vi "UI.vi"(9 "Event Registration Refnum in":refnum<event-registration>) -> ()   [LabVIEW 2019]
uses:
  Type Definitions/UI.ctl
  Type Definitions/UIOscillatorParam.ctl
  Type Definitions/Sub Oscillalator Type.ctl
  Type Definitions/UIADSRParam.ctl
  Type Definitions/UILowpassParam.ctl
  Type Definitions/UITremolo.ctl
  Type Definitions/DataInOut.ctl
panel:
  out "Waveform preview":waveform(dbl)(graph)
  in  "Input data":T1={"Play sound"=FALSE, "Stop Application"=FALSE, "Oscillator"={"Waveform Type"=enum."Sine Wave", "Frequency"=856.9737569249443, "Pulse Width"=50.10820125762328, "Sub oscillator"=enum."Off"}, "VCA"={"Volume"=49.9097556730832, "A"=50, "S"=100, "R"=50, "D"=50}, "Lowpass filter"={"On / Off"=FALSE, "Cutoff"=12290.454833178042}, "Tremolo"={"On / Off"=FALSE, "Frequency"=2.677004056526059, "Rate"=0.0}} {"Tremolo"."Rate" min=0.0 max=100.0 scale=0.0..1.0; "Tremolo"."Frequency" min=0.0 max=100.0 scale=0.0..25.0; "Lowpass filter"."Cutoff" min=0.0 max=100.0 scale=20.0..20000.0; "VCA"."D" scale=1.0..100.0; "VCA"."R" scale=1.0..100.0; "VCA"."S" scale=1.0..100.0; "VCA"."A" scale=1.0..100.0; "VCA"."Volume" min=0.0 max=100.0 scale=0.0..100.0; "Oscillator"."Pulse Width" min=0.0 max=100.0 scale=0.0..100.0; "Oscillator"."Frequency" min=0.0 max=100.0 scale=20.0..20000.0}
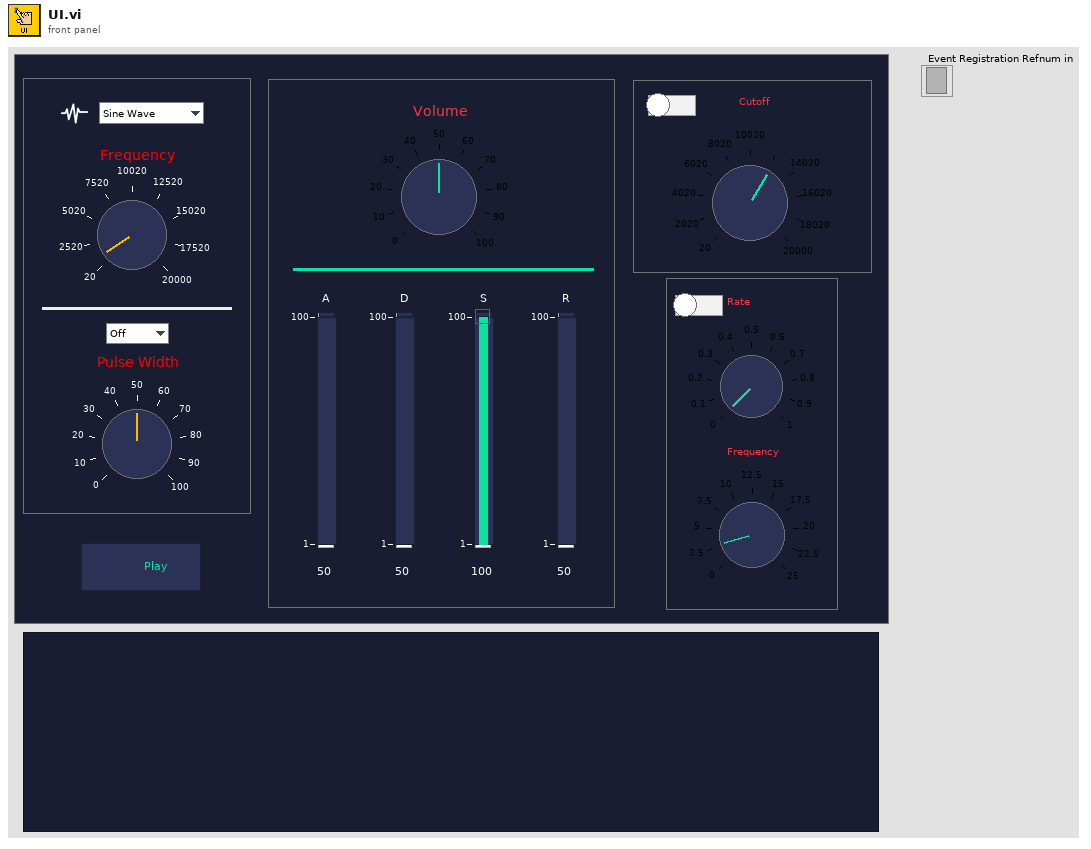
[diagram p1: front panel]
types:
  T1 = typedef "UI.ctl" = cluster{"Play sound":bool, "Stop Application":bool, "Oscillator":T2, "VCA":T4, "Lowpass filter":T5, "Tremolo":T6}
  T2 = typedef "UIOscillatorParam.ctl" = cluster{"Waveform Type":enum16{"Sine Wave", "Triangle Wave", "Square Wave", "Sawtooth Wave"}, "Frequency":dbl, "Pulse Width":dbl, "Sub oscillator":T3}
  T3 = typedef "Sub Oscillalator Type.ctl" = enum16{"Off", "One Octave", "Two Octaves"}
  T4 = typedef "UIADSRParam.ctl" = cluster{"Volume":dbl, "A":i8, "S":i8, "R":i8, "D":i8}
  T5 = typedef "UILowpassParam.ctl" = cluster{"On / Off":bool, "Cutoff":dbl}
  T6 = typedef "UITremolo.ctl" = cluster{"On / Off":bool, "Frequency":dbl, "Rate":dbl}
  T7 = typedef "DataInOut.ctl" = enum16{"Write", "Read"}
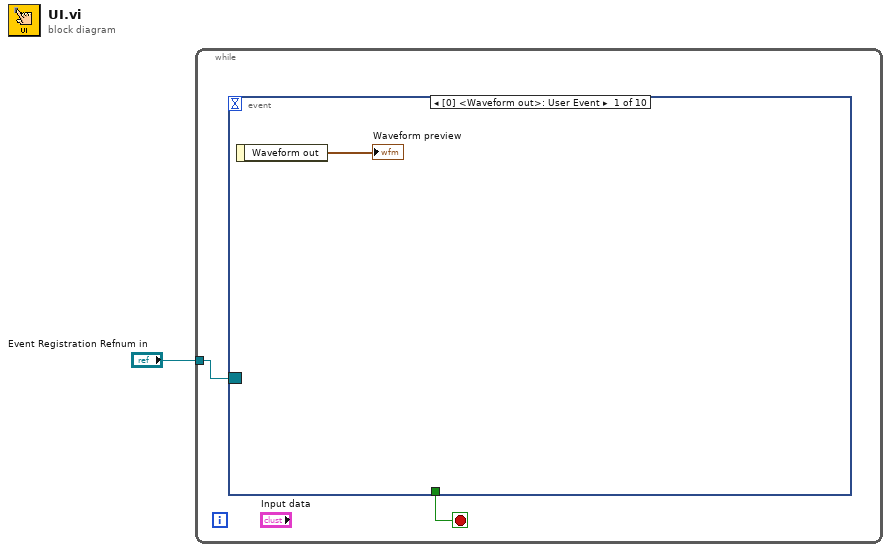
[diagram p0: block diagram]
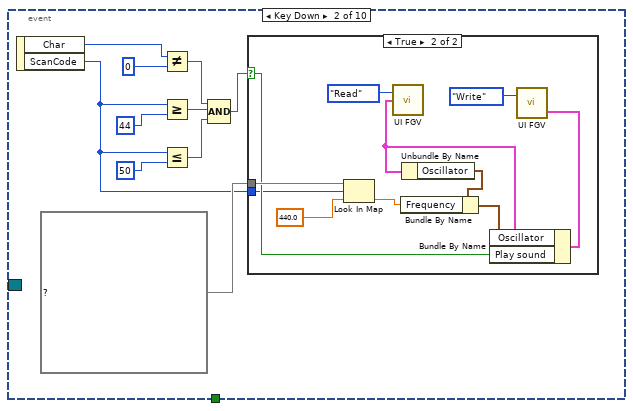
[diagram p2: hidden frame]
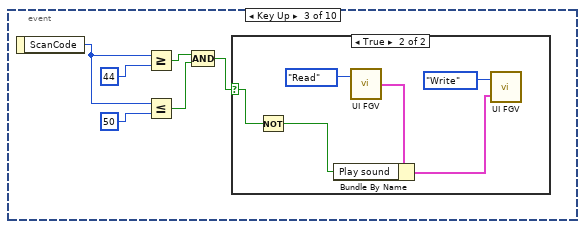
[diagram p4: hidden frame]
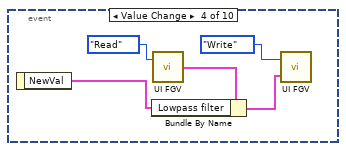
[diagram p6: hidden frame]
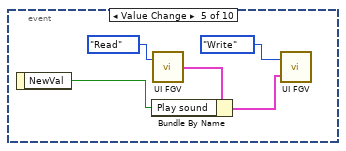
[diagram p7: hidden frame]
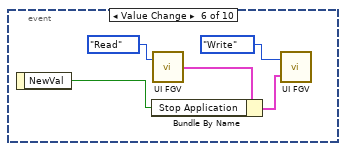
[diagram p8: hidden frame]
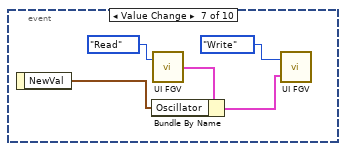
[diagram p9: hidden frame]
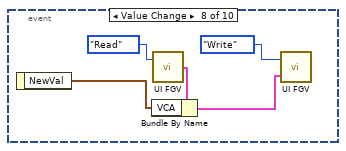
[diagram p10: hidden frame]
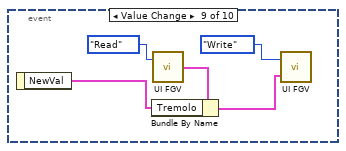
[diagram p11: hidden frame]
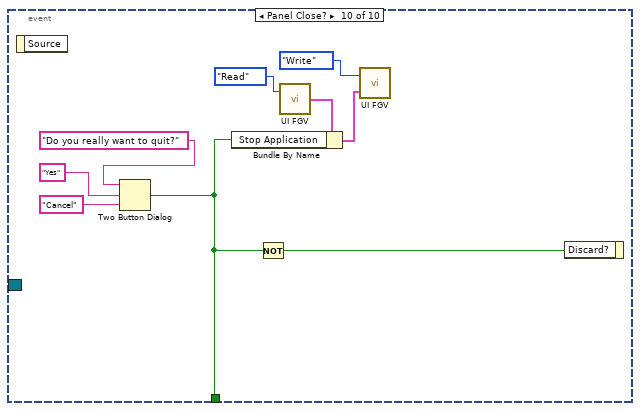
[diagram p12: hidden frame]
diagram:
  n1 = while "User Interface" {
    tunnel: "Event Registration Refnum in" -> [w3]
    stop <- w2 stop-if-true
    n2 = event shown="[0] <Waveform out>: User Event" {
      selector: w3 -> [_ _ _ _ _ _ _ _ _ _]
      dyn-events: _ -> [_ _ _ _ _ _ _ _ _ _]
      timeout: _ -> [_ _ _ _ _ _ _ _ _ _]
      tunnel: [_ _ _ _ _ _ _ _ _ w68] -> w2
      event User Event {
        n3 = event-data() -> ("Waveform out"=→"Waveform preview":waveform(dbl))  [unwired: 1 in]
      }
      event Key Down {
        n4 = event-data() -> ("Char"=w7:i16, "ScanCode"=w5:i16)  [unwired: 1 in]
        n5 = Not Equal?(x=w7, y=i16 0) -> (x != y?=w11:bool)
        n6 = Greater Or Equal?(x=w5, y=i16 44) -> (x >= y?=w10:bool)
        n7 = Less Or Equal?(x=w5, y=i16 50) -> (x <= y?=w9:bool)
        n8 = Compound Arithmetic op=AND(w11, w10, w9) -> (w6:bool)
        n9 = case shown="True" w6 {
          selector: w6 -> [_ w16]
          tunnel: map{i16, dbl} {44=261.6255653005986, 45=277.1826309768721, 46=293.66476791740763, 47=311.1269837220809, 48=329.62755691286986, 49=349.22823143300394, 50=369.9944227116344} ("Map") -> [_ w25]
          tunnel: w5 -> [_ w15]
          frame False {
          }
          frame True {
            n10 = Look In Map(map=w25, key=w15, default value=440.0) -> (value=w17:dbl)  [unwired: 1 out]
            n11 = call "UI FGV.vi"("Mode"=DataInOut."Read" ("Enum")) -> ("Data out"=w20:T1)  [unwired: 1 in]
            n12 = Unbundle By Name(w20) -> ("Oscillator"=w19:T2)
            n13 = Bundle By Name(cluster=w19, "Frequency"=w17) -> (w18:T2)
            n14 = Bundle By Name(cluster=w20, "Oscillator"=w18, "Play sound"=w16) -> (w21:T1)
            n15 = call "UI FGV.vi"("Data in"=w21, "Mode"=DataInOut."Write" ("Enum")) -> ()  [unwired: 1 out]
          }
        }
      }
      event Key Up {
        n16 = event-data() -> ("ScanCode"=w28:i16)  [unwired: 1 in]
        n17 = Greater Or Equal?(x=w28, y=i16 44) -> (x >= y?=w27:bool)
        n18 = Less Or Equal?(x=w28, y=i16 50) -> (x <= y?=w26:bool)
        n19 = Compound Arithmetic op=AND(w27, w26) -> (w31:bool)
        n20 = case shown="True" w31 {
          selector: w31 -> [_ w32]
          frame False {
          }
          frame True {
            n21 = Not(x=w32) -> (.not. x?=w35:bool)
            n22 = call "UI FGV.vi"("Mode"=DataInOut."Read" ("Enum")) -> ("Data out"=w34:T1)  [unwired: 1 in]
            n23 = Bundle By Name(cluster=w34, "Play sound"=w35) -> (w33:T1)
            n24 = call "UI FGV.vi"("Data in"=w33, "Mode"=DataInOut."Write" ("Enum")) -> ()  [unwired: 1 out]
          }
        }
      }
      event Value Change {
        n25 = event-data() -> ("NewVal"=w38:T5)  [unwired: 1 in]
        n26 = call "UI FGV.vi"("Mode"=DataInOut."Read" ("Enum")) -> ("Data out"=w42:T1)  [unwired: 1 in]
        n27 = Bundle By Name(cluster=w42, "Lowpass filter"=w38) -> (w41:T1)
        n28 = call "UI FGV.vi"("Data in"=w41, "Mode"=DataInOut."Write" ("Enum")) -> ()  [unwired: 1 out]
      }
      event Value Change {
        n29 = event-data() -> ("NewVal"=w43:bool)  [unwired: 1 in]
        n30 = call "UI FGV.vi"("Mode"=DataInOut."Read" ("Enum")) -> ("Data out"=w47:T1)  [unwired: 1 in]
        n31 = Bundle By Name(cluster=w47, "Play sound"=w43) -> (w46:T1)
        n32 = call "UI FGV.vi"("Data in"=w46, "Mode"=DataInOut."Write" ("Enum")) -> ()  [unwired: 1 out]
      }
      event Value Change {
        n33 = event-data() -> ("NewVal"=w48:bool)  [unwired: 1 in]
        n34 = call "UI FGV.vi"("Mode"=DataInOut."Read" ("Enum")) -> ("Data out"=w52:T1)  [unwired: 1 in]
        n35 = Bundle By Name(cluster=w52, "Stop Application"=w48) -> (w51:T1)
        n36 = call "UI FGV.vi"("Data in"=w51, "Mode"=DataInOut."Write" ("Enum")) -> ()  [unwired: 1 out]
      }
      event Value Change {
        n37 = event-data() -> ("NewVal"=w53:T2)  [unwired: 1 in]
        n38 = call "UI FGV.vi"("Mode"=DataInOut."Read" ("Enum")) -> ("Data out"=w57:T1)  [unwired: 1 in]
        n39 = Bundle By Name(cluster=w57, "Oscillator"=w53) -> (w56:T1)
        n40 = call "UI FGV.vi"("Data in"=w56, "Mode"=DataInOut."Write" ("Enum")) -> ()  [unwired: 1 out]
      }
      event Value Change {
        n41 = event-data() -> ("NewVal"=w58:T4)  [unwired: 1 in]
        n42 = call "UI FGV.vi"("Mode"=DataInOut."Read" ("Enum")) -> ("Data out"=w62:T1)  [unwired: 1 in]
        n43 = Bundle By Name(cluster=w62, "VCA"=w58) -> (w61:T1)
        n44 = call "UI FGV.vi"("Data in"=w61, "Mode"=DataInOut."Write" ("Enum")) -> ()  [unwired: 1 out]
      }
      event Value Change {
        n45 = event-data() -> ("NewVal"=w63:T6)  [unwired: 1 in]
        n46 = call "UI FGV.vi"("Mode"=DataInOut."Read" ("Enum")) -> ("Data out"=w67:T1)  [unwired: 1 in]
        n47 = Bundle By Name(cluster=w67, "Tremolo"=w63) -> (w66:T1)
        n48 = call "UI FGV.vi"("Data in"=w66, "Mode"=DataInOut."Write" ("Enum")) -> ()  [unwired: 1 out]
      }
      event Panel Close? {
        n49 = event-data() -> ()  [unwired: 1 in, 1 out]
        n50 = Two Button Dialog(message="Do you really want to quit?", 1:"Cancel", 2:"Yes") -> (T button?=w68:bool)
        n51 = Not(x=w68) -> (.not. x?=w69:bool)
        n52 = call "UI FGV.vi"("Mode"=DataInOut."Read" ("Enum")) -> ("Data out"=w72:T1)  [unwired: 1 in]
        n53 = Bundle By Name(cluster=w72, "Stop Application"=w68) -> (w73:T1)
        n54 = call "UI FGV.vi"("Data in"=w73, "Mode"=DataInOut."Write" ("Enum")) -> ()  [unwired: 1 out]
        n55 = event-data("Discard?"=w69) -> ()  [unwired: 1 in, 1 out]
      }
    }
  }
